vi "Align to Pos.vi"(10 "Robot Velocities In":T3={"X Velocity"=0.0, "Y Velocity"=0.0, "Rotational \nVelocity"=100.0}, 11 "Field Element":enum16{"Bump", "Shooter Shot", "Trench"}(ring)) -> (0 "Done?":bool, 2 "Robot Velocities Out":T3={"X Velocity"=1.7996659220144537, "Y Velocity"=0.5747831527820036, "Rotational \nVelocity"=100.0})   [LabVIEW 2025]
uses:
  swerve-template/Type Definitions/Data/Robot Velocities.ctl
  <vilib>/Rock Robotics/WPI/DriverStation/WPI_DriverStationAllianceInfo.ctl
  <vilib>/Rock Robotics/Network Tables/NT Read Numeric Array.vi
  Framework/Robot Global Data.vi
  <vilib>/addons/control/pid/pid.llb/PID (DBL).vi
  <vilib>/addons/control/pid/NI_PID_pid.lvlib
panel:
  out "Field Element 2":enum16{"Bump", "Shooter Shot", "Trench"}(ring)
  out "Current Pose":cluster{dbl, dbl}
  in  "PID gains":T1={"proportional gain (Kc)"=1.5, "integral time (Ti, min)"=0.0, "derivative time (Td, min)"=0.0} {"derivative time (Td, min)" format="%.3f"; "integral time (Ti, min)" format="%.3f"; "proportional gain (Kc)" format="%.3f"}
  in  "output range":cluster{"output high":dbl, "output low":dbl}={"output high"=5.0, "output low"=-5.0} {"output low" format="%.2f"; "output high" format="%.2f"}
  out "Cluster":cluster{"X":dbl, "Y":dbl}={"X"=8.2, "Y"=43.27}
  in  "Array":cluster{"X":dbl, "Y":dbl}[][](array[cluster])=[[{"X"=8.1, "Y"=20.897}, {"X"=1.7, "Y"=44.57}, {"X"=1.7, "Y"=44.57}], [{"X"=18.2, "Y"=20.897}, {"X"=18.2, "Y"=44.57}, {"X"=18.2, "Y"=44.57}], [{"X"=18.2, "Y"=33.37}, {"X"=18.2, "Y"=9.7}, {"X"=18.2, "Y"=9.7}], [{"X"=8.1, "Y"=33.37}, {"X"=8.6, "Y"=9.7}, {"X"=8.6, "Y"=9.7}]]
  out "Velocities OUT":T2(graph)={"X Velocity"=1.7996659220144537, "Y Velocity"=0.5747831527820036, "Rotational \nVelocity"=100.0}
  out "Tag IDs":dbl(graph)=2.0
  out "Correction":cluster{dbl, dbl}(graph)={1.7996659220144537, 0.5747831527820036}
  # "Shooter  Shot"
  # "Trench"
  # "Bump"
  # "Red Outpost"
  # "Red Depot"
  # "Blue Outpost"
  # "Blue Depot"
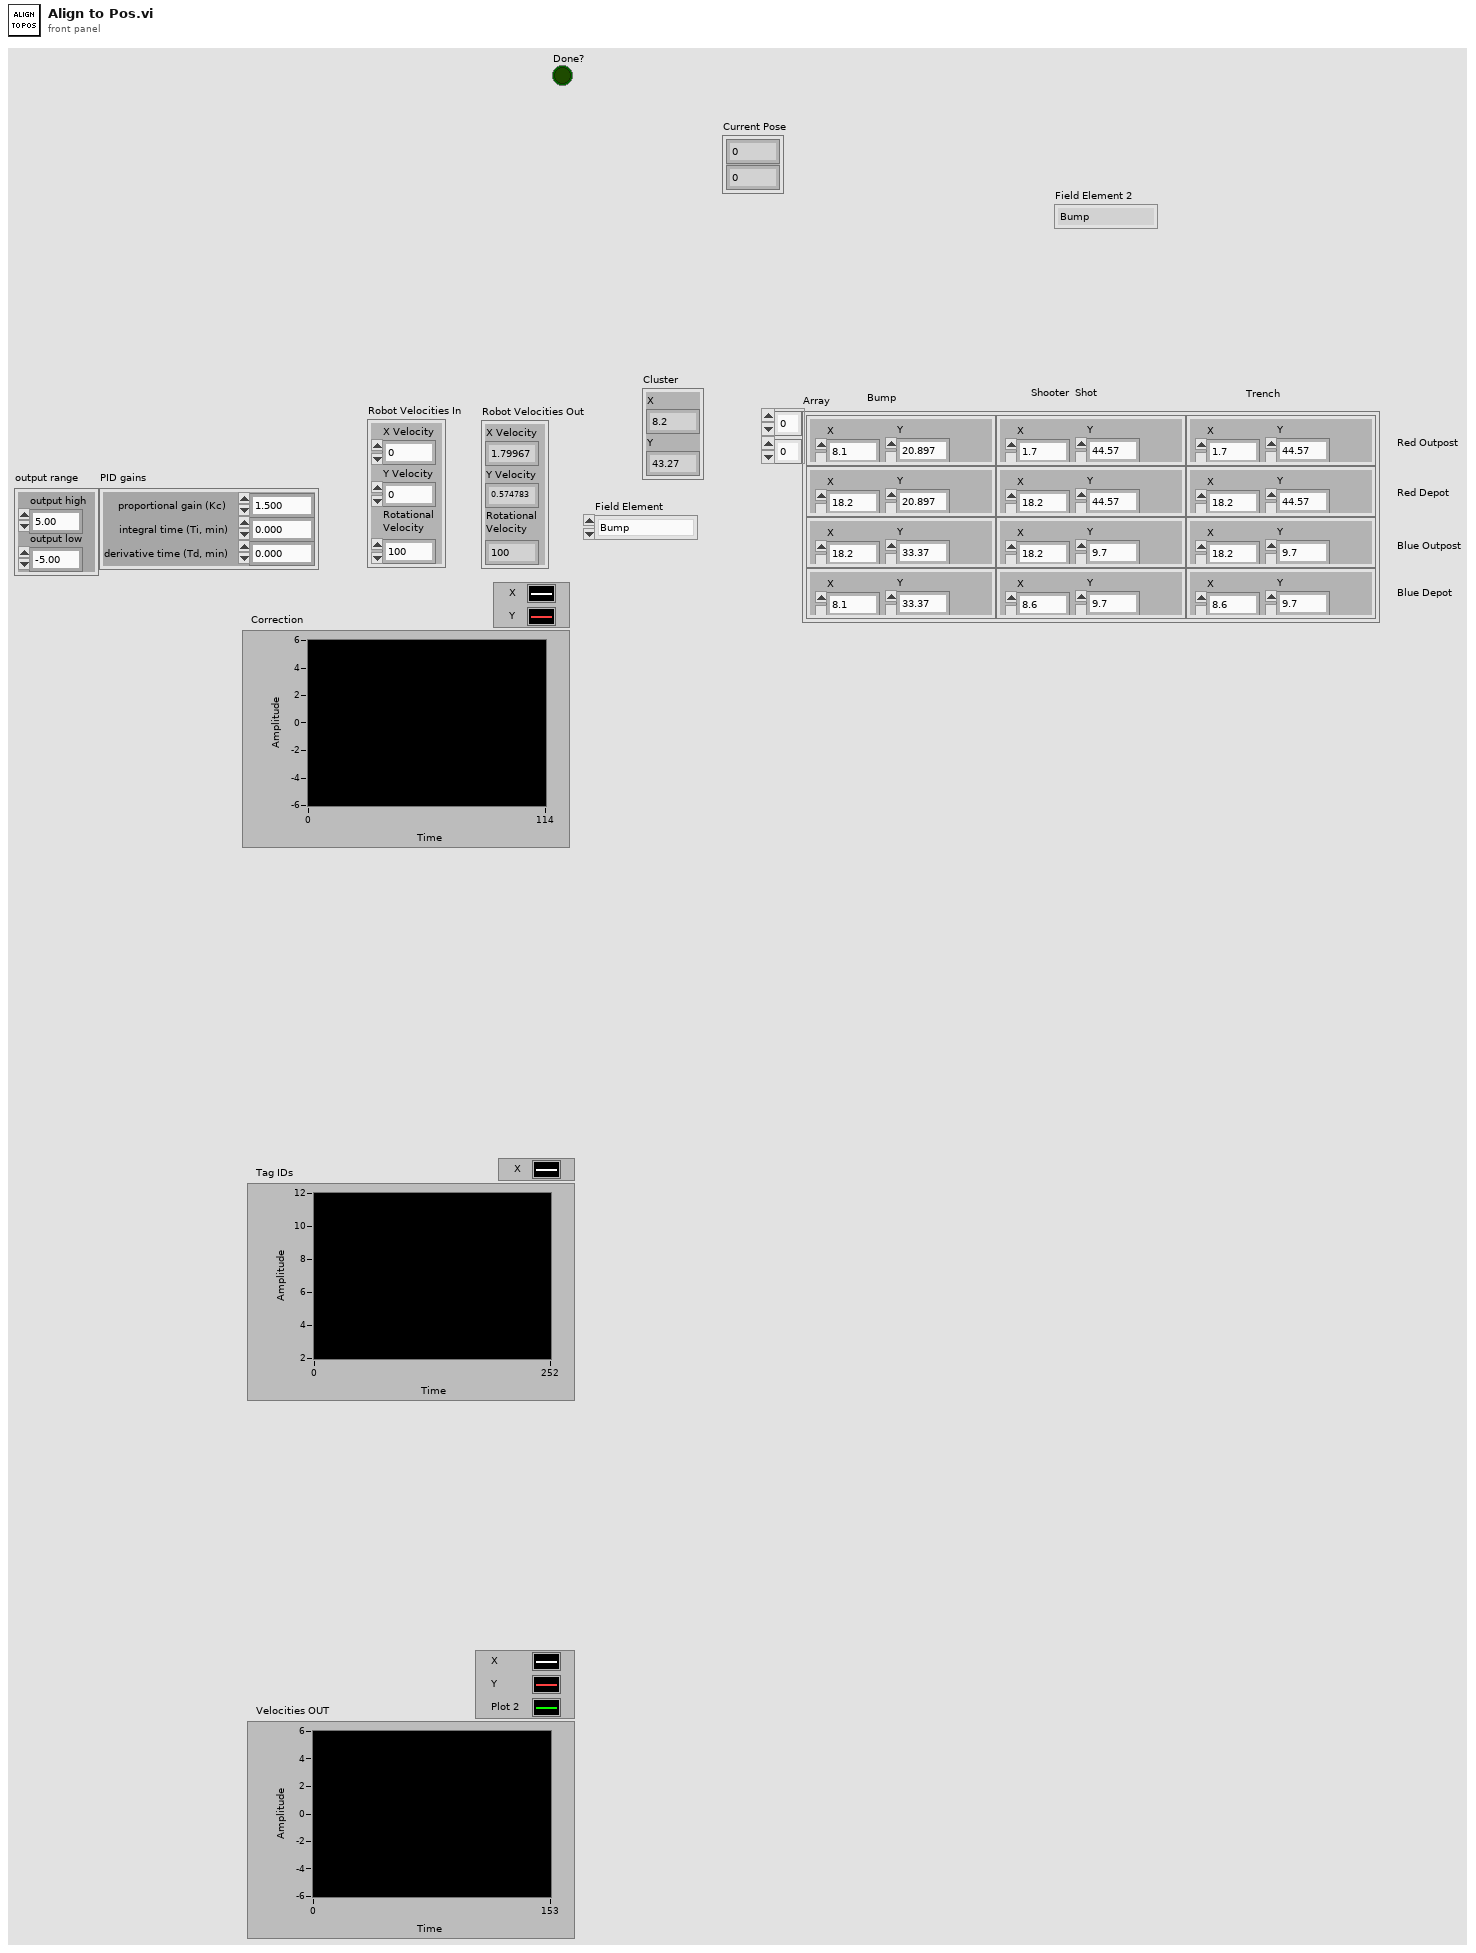
[diagram p1: front panel]
types:
  T1 = cluster{"proportional gain (Kc)":dbl, "integral time (Ti, min)":dbl, "derivative time (Td, min)":dbl}
  T2 = cluster{"X Velocity":dbl, "Y Velocity":dbl, "Rotational \nVelocity":dbl}
  T3 = typedef "Robot Velocities.ctl" = cluster{"X Velocity":dbl, "Y Velocity":dbl, "Rotational \nVelocity":dbl}
  T4 = typedef "WPI_DriverStationAllianceInfo.ctl" = enum16{"Red", "Blue", "Invalid"}
  T5 = typedef "Drive Conditions.ctl" = cluster{"Field Centric":bool, "BotPose Correction":bool, "Theta Align":bool, "Current Limit 50A(F) 60A(T)":bool, "Align to Field":cluster{"Align to Bump or Shoot":bool, "Field Element":enum16{"Bump", "Shooter Shot", "Trench"}}}
  T6 = cluster{bool, "Field Element":enum16{"Bump", "Shooter Shot", "Trench"}}
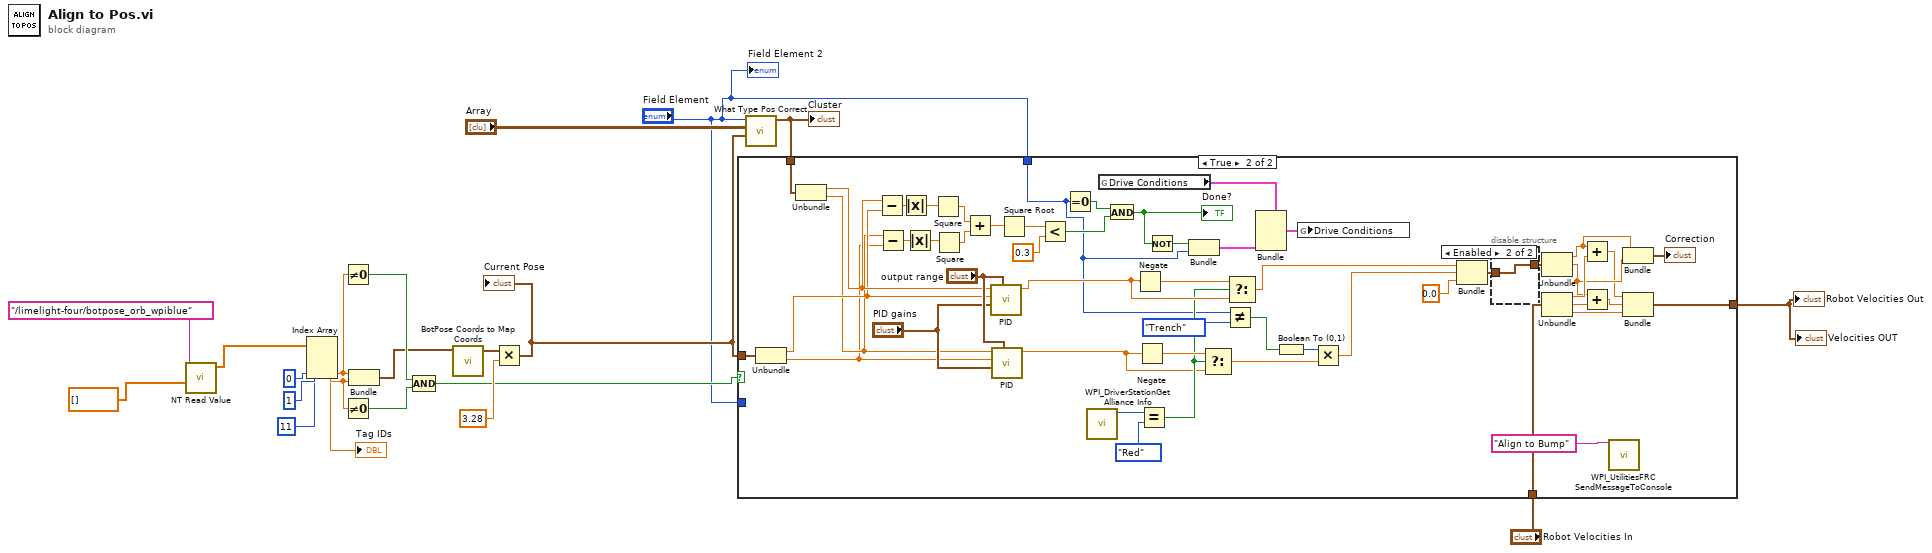
[diagram p0: block diagram]
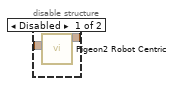
[diagram p3: hidden frame]
diagram:
  n1 = call-poly <vilib>:"NT Read Value.vi"("default value"=dbl[] [], "name"="/limelight-four/botpose_orb_wpiblue") -> ("value"=w20:dbl[])  [unwired: 7 in, 2 out]
  n2 = Index Array(array=w20, index #1=0 ("index"), index #2=1 ("index"), index #3=11 ("index")) -> (element #1=w15:dbl, element #2=w14:dbl, element #3=→"Tag IDs":dbl)
  n3 = Not Equal To 0?(x=w15) -> (x != 0?=w17:bool)
  n4 = Not Equal To 0?(x=w14) -> (x != 0?=w16:bool)
  n5 = Bundle("Numeric"=w15, "Numeric"=w14) -> (w8:cluster{"Numeric":dbl, "Numeric":dbl})  [unwired: 1 in]
  n6 = Compound Arithmetic op=AND(w17, w16) -> (w2:bool)
  n7 = call "BotPose Coords to Map Coords.vi"("Point In"=w8) -> ("Point Out"=w6:cluster{dbl, dbl})  [unwired: 10 in]
  n8 = Multiply(x=w6, y=3.28) -> (x*y=w3:cluster{dbl, dbl})
  "Current Pose" <- w3
  n9 = call "What Type Pos Correct.vi"("Point In"=w3, "Array"="Array", "Field Element"="Field Element") -> ("Cluster out"=w7:cluster{"X":dbl, "Y":dbl})  [unwired: 8 in]
  "Cluster" <- w7
  n10 = case shown="True" w2 {
    tunnel: w3 -> [_ w60]
    tunnel: [w22 w64] -> w11
    tunnel: "Robot Velocities In" -> [w22 w74]
    tunnel: w7 -> [_ w62]
    tunnel: "Field Element" -> [_ _]
    tunnel: "Field Element" -> [_ w23]
    frame False {
    }
    frame True {
      n11 = Unbundle(w60) -> (w57:dbl, w55:dbl)
      n12 = Unbundle(w62) -> ("X"=w58:dbl, "Y"=w56:dbl)
      n13 = Subtract(x=w58, y=w57) -> (x-y=w53:dbl)
      n14 = Subtract(x=w56, y=w55) -> (x-y=w54:dbl)
      n15 = Absolute Value(x=w53) -> (abs(x)=w52:dbl)
      n16 = Absolute Value(x=w54) -> (abs(x)=w51:dbl)
      n17 = Square(x=w52) -> (x^2=w49:dbl)
      n18 = Square(x=w51) -> (x^2=w50:dbl)
      n19 = Add(x=w49, y=w50) -> (x+y=w48:dbl)
      n20 = call-poly <vilib>:"PID.vi"("output range"="output range", "PID gains"="PID gains", "process variable"=w57, "setpoint"=w58) -> ("output"=w40:dbl)  [unwired: 6 in, 1 out]
      n21 = call-poly <vilib>:"PID.vi"("output range"="output range", "PID gains"="PID gains", "process variable"=w55, "setpoint"=w56) -> ("output"=w36:dbl)  [unwired: 6 in, 1 out]
      n22 = Square Root(x=w48) -> (sqrt(x)=w47:dbl)
      n23 = Less?(x=w47, y=0.3) -> (x < y?=w29:bool)
      n24 = Equal To 0?(x=w23) -> (x = 0?=w30:bool)
      n25 = call <vilib>:"WPI_DriverStationGet Alliance Info.vi"() -> ("Alliance"=w45:T4)  [unwired: 6 in, 5 out]
      n26 = global read "Robot Global Data.vi" "Drive Conditions"() -> (w34:T5)
      n27 = And(x=w30, y=w29) -> (x .and. y?=w35:bool)
      "Done?" <- w35
      n28 = Negate(x=w40) -> (-x=w41:dbl)
      n29 = Negate(x=w36) -> (-x=w43:dbl)
      n30 = Equal?(x=w45, y=WPI_DriverStationAllianceInfo."Red") -> (x = y?=w38:bool)
      n31 = Not(x=w35) -> (.not. x?=w32:bool)
      n32 = Bundle(w32, "Field Element"=w23) -> (w31:T6)  [unwired: 1 in]
      n33 = Select(t=w43, s=w38, f=w36) -> (s? t:f=w25:dbl)
      n34 = Not Equal?(x=w23, y=enum16{"Bump", "Shooter Shot", "Trench"}."Trench") -> (x != y?=w28:bool)
      n35 = Select(t=w41, s=w38, f=w40) -> (s? t:f=w39:dbl)
      n36 = Bundle(cluster=w34, "Align to Field"=w31) -> (w33:T5)  [unwired: 4 in]
      n37 = Boolean To (0,1)(Boolean=w28) -> (0, 1=w26:i16)
      n38 = global write "Robot Global Data.vi" "Drive Conditions"(w33) -> ()
      n39 = Multiply(x=w26, y=w25) -> (x*y=w24:dbl)
      n40 = Bundle("output"=w39, w24, 0.0) -> (w42:cluster{"output":dbl, dbl, dbl})  [unwired: 1 in]
      n41 = disable-structure shown="Enabled" {
        disable-tunnel: [w76 w77] -> w72
        disable-tunnel: w42 -> [w75 w77]
        frame Disabled {
          n42 = call "Pigeon2 Robot Centric.vi"("Robot Centric Velocities"=w75) -> ("Field Centric Velocities"=w76:T3)  [unwired: 10 in]
        }
        frame Enabled {
        }
      }
      n43 = Unbundle(w72) -> ("output"=w66:dbl, w65:dbl)  [unwired: 1 out]
      n44 = Unbundle(w74) -> ("X Velocity"=w67:dbl, "Y Velocity"=w70:dbl, "Rotational \nVelocity"=w73:dbl)
      n45 = Add(x=w66, y=w67) -> (x+y=w63:dbl)
      n46 = Add(x=w65, y=w70) -> (x+y=w69:dbl)
      n47 = call <vilib>:"WPI_UtilitiesFRC SendMessageToConsole.vi"("Message"="Align to Bump") -> ()  [unwired: 14 in, 1 out]
      n48 = Bundle("output"=w66, w65) -> (→"Correction":cluster{"output":dbl, dbl})  [unwired: 1 in]
      n49 = Bundle(w63, w69, "Rotational \nVelocity"=w73) -> (w64:cluster{dbl, dbl, "Rotational \nVelocity":dbl})  [unwired: 1 in]
    }
  }
  "Robot Velocities Out" <- w11
  "Velocities OUT" <- w11
  "Field Element 2" <- "Field Element"
